vi "Read Power Supply classes.vi"(11 "Measurements in":refnum<class "Measurement.lvclass">) -> (2 "Power Supply classes":refnum<class "Power Supply.lvclass">[](array[class]), 3 "Measurements out":refnum<class "Measurement.lvclass">)   [LabVIEW 2020, in "Measurement.lvclass"]
uses:
  Measurement.lvclass
  Instruments/Power Supply/Power Supply.lvclass
  Measurement.lvclass/Measurement.ctl
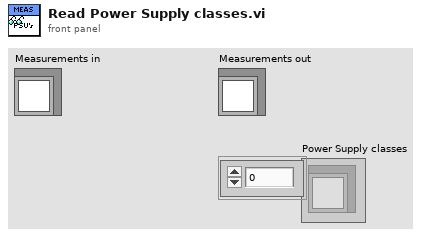
[diagram p1: front panel]
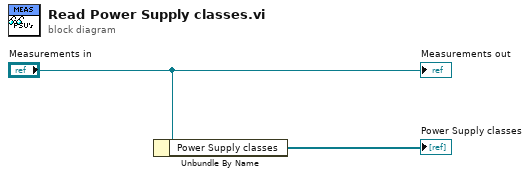
[diagram p0: block diagram]
diagram:
  n1 = Unbundle By Name("Measurements in") -> ("Power Supply classes"=→"Power Supply classes":refnum<class "Power Supply.lvclass">[])
  "Measurements out" <- "Measurements in"
